vi "EOL Digital IO Status.vi"() -> ()   [LabVIEW 2018]
uses:
  05.UserVI's/type defs/EOL Global Digital Output Cluster Control.ctl
  05.UserVI's/type defs/EOL Global Digital Output Control.ctl
  05.UserVI's/type defs/EOL Global Digital Input Control.ctl
panel:
  in  "Tab Control":enum32{"Digital I/O", "RSLinx Tags"}(tab)
  out "Digital Inputs":T2(array[cluster])=[{"Status"=FALSE, "EOL Global Digital Input Control"=enum."Dev2/port0/line0"}, {"Status"=FALSE, "EOL Global Digital Input Control"=enum."Dev2/port0/line1"}, {"Status"=FALSE, "EOL Global Digital Input Control"=enum."Dev2/port0/line2"}, {"Status"=FALSE, "EOL Global Digital Input Control"=enum."Dev2/port0/line3"}, {"Status"=FALSE, "EOL Global Digital Input Control"=enum."Dev2/port0/line4"}, {"Status"=FALSE, "EOL Global Digital Input Control"=enum."Dev2/port0/line5"}, {"Status"=FALSE, "EOL Global Digital Input Control"=enum."Dev2/port0/line6"}, {"Status"=FALSE, "EOL Global Digital Input Control"=enum."Dev2/port0/line7"}, {"Status"=FALSE, "EOL Global Digital Input Control"=enum."Dev2/port1/line0"}, {"Status"=FALSE, "EOL Global Digital Input Control"=enum."Dev2/port1/line1"}, {"Status"=FALSE, "EOL Global Digital Input Control"=enum."Dev2/port1/line2"}, {"Status"=FALSE, "EOL Global Digital Input Control"=enum."Dev2/port1/line3"}, {"Status"=FALSE, "EOL Global Digital Input Control"=enum."Dev2/port1/line4"}, {"Status"=FALSE, "EOL Global Digital Input Control"=enum."Dev2/port1/line5"}, {"Status"=FALSE, "EOL Global Digital Input Control"=enum."Dev2/port1/line6"}, {"Status"=FALSE, "EOL Global Digital Input Control"=enum."Dev2/port1/line7"}, {"Status"=FALSE, "EOL Global Digital Input Control"=enum."Dev2/port2/line0"}, {"Status"=FALSE, "EOL Global Digital Input Control"=enum."Dev2/port2/line1"}, {"Status"=FALSE, "EOL Global Digital Input Control"=enum."Dev2/port2/line2"}, {"Status"=FALSE, "EOL Global Digital Input Control"=enum."Dev2/port2/line3"}, {"Status"=FALSE, "EOL Global Digital Input Control"=enum."Dev2/port2/line4"}, {"Status"=FALSE, "EOL Global Digital Input Control"=enum."Dev2/port2/line5"}, {"Status"=FALSE, "EOL Global Digital Input Control"=enum."Dev2/port2/line6"}, {"Status"=FALSE, "EOL Global Digital Input Control"=enum."Dev2/port2/line7"}, {"Status"=FALSE, "EOL Global Digital Input Control"=enum."Prerun Start Test"}, {"Status"=FALSE, "EOL Global Digital Input Control"=enum."Prerun Abort Test"}, {"Status"=FALSE, "EOL Global Digital Input Control"=enum."Audit Start Test"}, {"Status"=FALSE, "EOL Global Digital Input Control"=enum."Audit Abort Test"}, {"Status"=FALSE, "EOL Global Digital Input Control"=enum."Dev2/port3/line4"}, {"Status"=FALSE, "EOL Global Digital Input Control"=enum."Dev2/port3/line5"}, {"Status"=FALSE, "EOL Global Digital Input Control"=enum."Breakin Start Test"}, {"Status"=FALSE, "EOL Global Digital Input Control"=enum."Breakin Abort Test"}]
  out "Digital Output Status":T3[](array[typedef])=[{"Status"=FALSE, "Global DO Ch"=enum."Battery"}, {"Status"=FALSE, "Global DO Ch"=enum."Battery"}, {"Status"=FALSE, "Global DO Ch"=enum."Battery"}, {"Status"=FALSE, "Global DO Ch"=enum."Battery"}, {"Status"=FALSE, "Global DO Ch"=enum."Battery"}, {"Status"=FALSE, "Global DO Ch"=enum."Battery"}, {"Status"=FALSE, "Global DO Ch"=enum."Battery"}, {"Status"=FALSE, "Global DO Ch"=enum."Battery"}, {"Status"=FALSE, "Global DO Ch"=enum."Battery"}, {"Status"=FALSE, "Global DO Ch"=enum."Battery"}, {"Status"=FALSE, "Global DO Ch"=enum."Battery"}, {"Status"=FALSE, "Global DO Ch"=enum."Battery"}, {"Status"=FALSE, "Global DO Ch"=enum."Battery"}, {"Status"=FALSE, "Global DO Ch"=enum."Battery"}, {"Status"=FALSE, "Global DO Ch"=enum."Battery"}, {"Status"=FALSE, "Global DO Ch"=enum."Battery"}, {"Status"=FALSE, "Global DO Ch"=enum."Battery"}, {"Status"=FALSE, "Global DO Ch"=enum."Battery"}, {"Status"=FALSE, "Global DO Ch"=enum."Battery"}, {"Status"=FALSE, "Global DO Ch"=enum."Battery"}, {"Status"=FALSE, "Global DO Ch"=enum."Battery"}, {"Status"=FALSE, "Global DO Ch"=enum."Battery"}, {"Status"=FALSE, "Global DO Ch"=enum."Battery"}, {"Status"=FALSE, "Global DO Ch"=enum."Battery"}, {"Status"=FALSE, "Global DO Ch"=enum."Battery"}, {"Status"=FALSE, "Global DO Ch"=enum."Battery"}, {"Status"=FALSE, "Global DO Ch"=enum."Battery"}, {"Status"=FALSE, "Global DO Ch"=enum."Battery"}, {"Status"=FALSE, "Global DO Ch"=enum."Battery"}, {"Status"=FALSE, "Global DO Ch"=enum."Battery"}, {"Status"=FALSE, "Global DO Ch"=enum."Battery"}, {"Status"=FALSE, "Global DO Ch"=enum."Battery"}, {"Status"=FALSE, "Global DO Ch"=enum."Battery"}, {"Status"=FALSE, "Global DO Ch"=enum."Battery"}, {"Status"=FALSE, "Global DO Ch"=enum."Battery"}, {"Status"=FALSE, "Global DO Ch"=enum."Battery"}, {"Status"=FALSE, "Global DO Ch"=enum."Battery"}, {"Status"=FALSE, "Global DO Ch"=enum."Battery"}, {"Status"=FALSE, "Global DO Ch"=enum."Battery"}, {"Status"=FALSE, "Global DO Ch"=enum."Battery"}, {"Status"=FALSE, "Global DO Ch"=enum."Battery"}, {"Status"=FALSE, "Global DO Ch"=enum."Battery"}, {"Status"=FALSE, "Global DO Ch"=enum."Battery"}, {"Status"=FALSE, "Global DO Ch"=enum."Battery"}, {"Status"=FALSE, "Global DO Ch"=enum."Battery"}, {"Status"=FALSE, "Global DO Ch"=enum."Battery"}, {"Status"=FALSE, "Global DO Ch"=enum."Battery"}, {"Status"=FALSE, "Global DO Ch"=enum."Battery"}, {"Status"=FALSE, "Global DO Ch"=enum."Battery"}, {"Status"=FALSE, "Global DO Ch"=enum."Battery"}, {"Status"=FALSE, "Global DO Ch"=enum."Battery"}, {"Status"=FALSE, "Global DO Ch"=enum."Battery"}, {"Status"=FALSE, "Global DO Ch"=enum."Battery"}, {"Status"=FALSE, "Global DO Ch"=enum."Battery"}, {"Status"=FALSE, "Global DO Ch"=enum."Battery"}, {"Status"=FALSE, "Global DO Ch"=enum."Battery"}, {"Status"=FALSE, "Global DO Ch"=enum."Battery"}, {"Status"=FALSE, "Global DO Ch"=enum."Battery"}, {"Status"=FALSE, "Global DO Ch"=enum."Battery"}, {"Status"=FALSE, "Global DO Ch"=enum."Battery"}, {"Status"=FALSE, "Global DO Ch"=enum."Battery"}, {"Status"=FALSE, "Global DO Ch"=enum."Battery"}, {"Status"=FALSE, "Global DO Ch"=enum."Battery"}, {"Status"=FALSE, "Global DO Ch"=enum."Battery"}, {"Status"=FALSE, "Global DO Ch"=enum."Battery"}, {"Status"=FALSE, "Global DO Ch"=enum."Battery"}, {"Status"=FALSE, "Global DO Ch"=enum."Battery"}, {"Status"=FALSE, "Global DO Ch"=enum."Battery"}, {"Status"=FALSE, "Global DO Ch"=enum."Battery"}, {"Status"=FALSE, "Global DO Ch"=enum."Battery"}, {"Status"=FALSE, "Global DO Ch"=enum."Battery"}, {"Status"=FALSE, "Global DO Ch"=enum."Battery"}, {"Status"=FALSE, "Global DO Ch"=enum."Battery"}, {"Status"=FALSE, "Global DO Ch"=enum."Battery"}, {"Status"=FALSE, "Global DO Ch"=enum."Battery"}, {"Status"=FALSE, "Global DO Ch"=enum."Battery"}, {"Status"=FALSE, "Global DO Ch"=enum."Battery"}, {"Status"=FALSE, "Global DO Ch"=enum."Battery"}, {"Status"=FALSE, "Global DO Ch"=enum."Battery"}, {"Status"=FALSE, "Global DO Ch"=enum."Battery"}, {"Status"=FALSE, "Global DO Ch"=enum."Battery"}, {"Status"=FALSE, "Global DO Ch"=enum."Battery"}, {"Status"=FALSE, "Global DO Ch"=enum."Battery"}, {"Status"=FALSE, "Global DO Ch"=enum."Battery"}, {"Status"=FALSE, "Global DO Ch"=enum."Battery"}, {"Status"=FALSE, "Global DO Ch"=enum."Battery"}, {"Status"=FALSE, "Global DO Ch"=enum."Battery"}, {"Status"=FALSE, "Global DO Ch"=enum."Battery"}, {"Status"=FALSE, "Global DO Ch"=enum."Battery"}, {"Status"=FALSE, "Global DO Ch"=enum."Battery"}, {"Status"=FALSE, "Global DO Ch"=enum."Battery"}, {"Status"=FALSE, "Global DO Ch"=enum."Battery"}, {"Status"=FALSE, "Global DO Ch"=enum."Battery"}, {"Status"=FALSE, "Global DO Ch"=enum."Battery"}, {"Status"=FALSE, "Global DO Ch"=enum."Battery"}, {"Status"=FALSE, "Global DO Ch"=enum."Battery"}, {"Status"=FALSE, "Global DO Ch"=enum."Battery"}, {"Status"=FALSE, "Global DO Ch"=enum."Battery"}, {"Status"=FALSE, "Global DO Ch"=enum."Battery"}, {"Status"=FALSE, "Global DO Ch"=enum."Battery"}, {"Status"=FALSE, "Global DO Ch"=enum."Battery"}, {"Status"=FALSE, "Global DO Ch"=enum."Battery"}, {"Status"=FALSE, "Global DO Ch"=enum."Battery"}, {"Status"=FALSE, "Global DO Ch"=enum."Battery"}, {"Status"=FALSE, "Global DO Ch"=enum."Battery"}, {"Status"=FALSE, "Global DO Ch"=enum."Battery"}, {"Status"=FALSE, "Global DO Ch"=enum."Battery"}, {"Status"=FALSE, "Global DO Ch"=enum."Battery"}, {"Status"=FALSE, "Global DO Ch"=enum."Battery"}, {"Status"=FALSE, "Global DO Ch"=enum."Battery"}, {"Status"=FALSE, "Global DO Ch"=enum."Battery"}, {"Status"=FALSE, "Global DO Ch"=enum."Battery"}, {"Status"=FALSE, "Global DO Ch"=enum."Battery"}, {"Status"=FALSE, "Global DO Ch"=enum."Battery"}, {"Status"=FALSE, "Global DO Ch"=enum."Battery"}, {"Status"=FALSE, "Global DO Ch"=enum."Battery"}, {"Status"=FALSE, "Global DO Ch"=enum."Battery"}, {"Status"=FALSE, "Global DO Ch"=enum."Battery"}, {"Status"=FALSE, "Global DO Ch"=enum."Battery"}, {"Status"=FALSE, "Global DO Ch"=enum."Battery"}, {"Status"=FALSE, "Global DO Ch"=enum."Battery"}, {"Status"=FALSE, "Global DO Ch"=enum."Battery"}, {"Status"=FALSE, "Global DO Ch"=enum."Battery"}, {"Status"=FALSE, "Global DO Ch"=enum."Battery"}, {"Status"=FALSE, "Global DO Ch"=enum."Battery"}, {"Status"=FALSE, "Global DO Ch"=enum."Battery"}, {"Status"=FALSE, "Global DO Ch"=enum."Battery"}, {"Status"=FALSE, "Global DO Ch"=enum."Battery"}]
  out "RSLinx Read String":cluster{"Tag String":string, "String":string}[](array[cluster])
  out "RSLinx Read Boolean":cluster{"Tag String":string, "Boolean":bool}[](array[cluster])
  in  "Exit":bool
  # "Digital I/O Status"
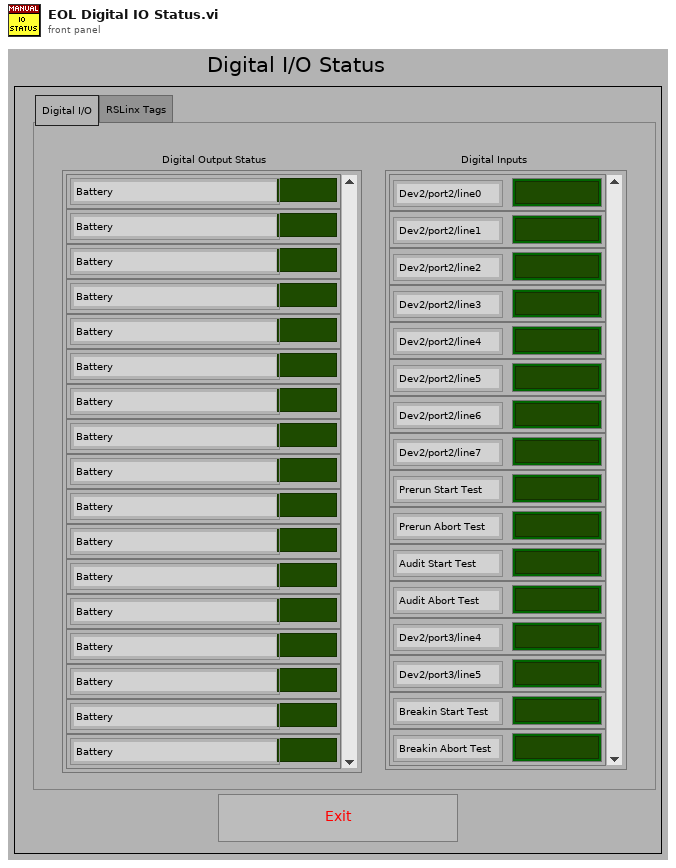
[diagram p1: front panel]
types:
  T1 = typedef "EOL Global Digital Input Control.ctl" = enum16{"Dev2/port0/line0", "Dev2/port0/line1", "Dev2/port0/line2", "Dev2/port0/line3", "Dev2/port0/line4", "Dev2/port0/line5", "Dev2/port0/line6", "Dev2/port0/line7", "Dev2/port1/line0", "Dev2/port1/line1", "Dev2/port1/line2", "Dev2/port1/line3", "Dev2/port1/line4", "Dev2/port1/line5", "Dev2/port1/line6", "Dev2/port1/line7", "Dev2/port2/line0", "Dev2/port2/line1", "Dev2/port2/line2", "Dev2/port2/line3", "Dev2/port2/line4", "Dev2/port2/line5", "Dev2/port2/line6", "Dev2/port2/line7", "Prerun Start Test", "Prerun Abort Test", "Audit Start Test", "Audit Abort Test", "Dev2/port3/line4", "Dev2/port3/line5", "Breakin Start Test", "Breakin Abort Test", "Not Implemented"}
  T2 = cluster{"Status":bool, "EOL Global Digital Input Control":T1}[]
  T3 = typedef "EOL Global Digital Output Cluster Control.ctl" = cluster{"Status":bool, "Global DO Ch":T4}
  T4 = typedef "EOL Global Digital Output Control.ctl" = enum16{"Battery", "IGN High", "IGN Low", "LIN", "CAN", "Switch 1", "Switch 2", "Switch 3", "Switch 4", "Switch 5", "Switch 6", "Glass Analog Switch 1", "Glass Analog Switch 2", "Glass Analog Switch 3", "Glass Analog Switch 4", "Sunshade Analog Switch 1", "Sunshade Analog Switch 2", "Sunshade Analog Switch 3", "Sunshade Analog Switch 4", "Glass Motor Relay 1", "Glass Motor Relay 2", "Sunshade Motor Relay 1", "Sunshade Motor Relay 2"}
  T5 = cluster{"RSLinx Write Boolean Names":string[], "RSLinx Write Boolean Tags":i32[], "RSLinx Write String Names":string[], "RSLinx Write String Tags":i32[], "RSLinx Read Boolean Names":string[], "RSLinx Read Boolean Tags":i32[], "RSLinx Read String Names":string[], "RSLinx Read String Tags":i32[], "Digital Output Array":T3[]}
  T6 = enum16{"Init", "Write", "Write All", "Clear All", "Stop", "Read"}
  T7 = cluster{"Status":bool, "EOL Global Digital Input Control":T1}
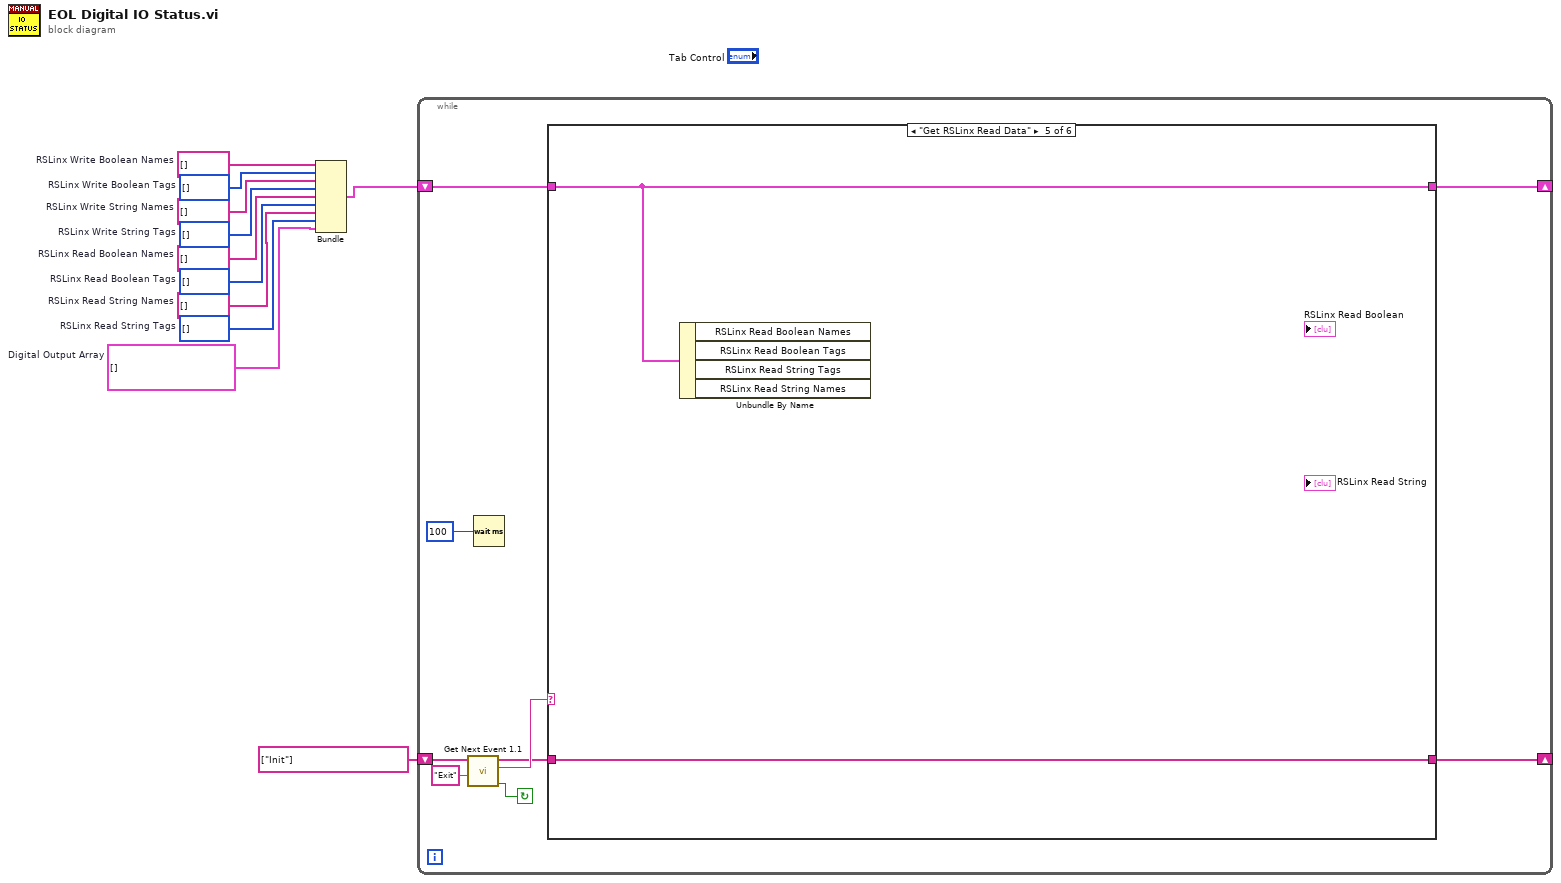
[diagram p0: block diagram]
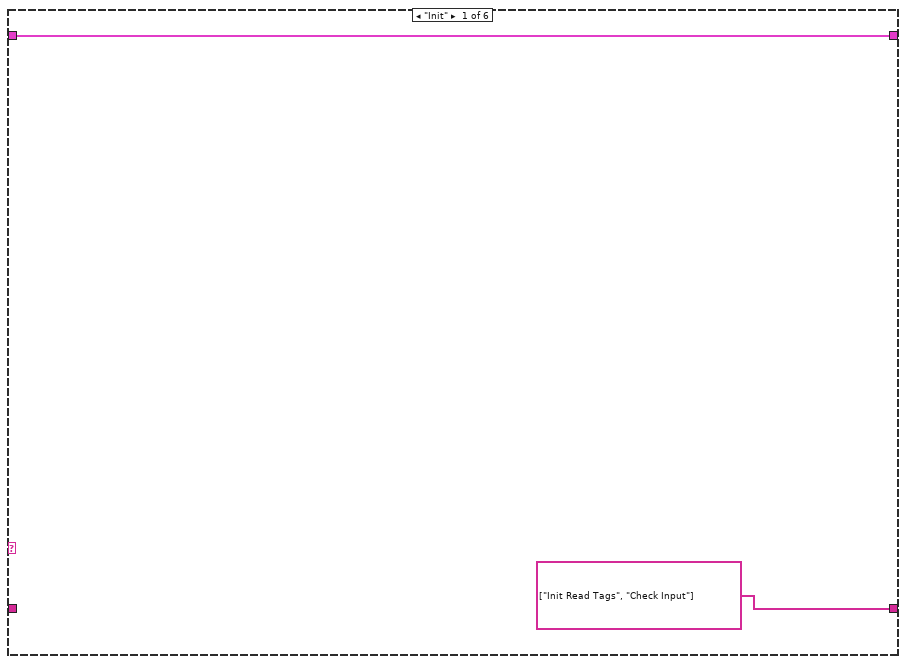
[diagram p2: hidden frame]
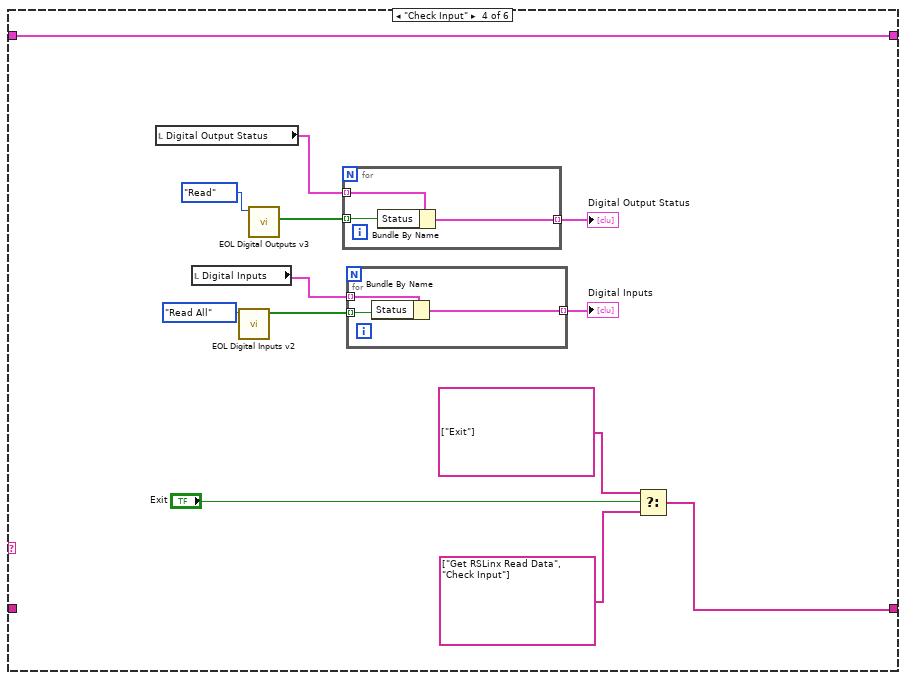
[diagram p5: hidden frame]
diagram:
  w1 = T3[] []  # Digital Output Array
  w5 = string[] []  # RSLinx Read String Names
  w4 = i32[] []  # RSLinx Read String Tags
  w7 = string[] []  # RSLinx Read Boolean Names
  w6 = i32[] []  # RSLinx Read Boolean Tags
  w9 = string[] []  # RSLinx Write String Names
  w8 = i32[] []  # RSLinx Write String Tags
  w11 = string[] []  # RSLinx Write Boolean Names
  w10 = i32[] []  # RSLinx Write Boolean Tags
  n1 = Bundle("RSLinx Write Boolean Names"=w11, "RSLinx Write Boolean Tags"=w10, "RSLinx Write String Names"=w9, "RSLinx Write String Tags"=w8, "RSLinx Read Boolean Names"=w7, "RSLinx Read Boolean Tags"=w6, "RSLinx Read String Names"=w5, "RSLinx Read String Tags"=w4, "Digital Output Array"=w1) -> (w3:T5)  [unwired: 1 in]
  n2 = while {
    shift-right: [w18] -> _
    shift-left: w3 -> [w19]
    shift-right: [w14] -> _
    shift-left: string[] ["Init"] ("event queue out") -> [w13]
    stop <- w12 continue-if-true
    n3 = call "Get Next Event 1.1.vi"("Exit Event"="Exit", "event queue in"=w13) -> ("Condition (Exit:F)"=w12:bool, "next event"=w16:string, "event queue out"=w15:string[])  [unwired: 6 in, 1 out]
    n4 = Wait (ms)(milliseconds to wait=u32 100) -> ()  [unwired: 1 out]
    n5 = case shown="\"Get RSLinx Read Data\"" w16 {
      tunnel: w19 -> [w22 w23 w25 w34 w47 w49]
      tunnel: [w22 w23 w25 w34 w47 w49] -> w18
      tunnel: w15 -> [_ w24 w26 _ w46 w48]
      tunnel: [string[] ["Init Read Tags", "Check Input"] ("event queue out") w24 w26 w27 w46 w48] -> w14
      frame "Init" {
      }
      frame "Init Read Tags" {
      }
      frame "Init Write Tags" {
      }
      frame "Check Input" {
        n6 = local read "Digital Output Status"() -> (w33:T3[])
        n7 = local read "Digital Inputs"() -> (w31:T2)
        n8 = call "EOL Digital Inputs v2.vi"("Mode"=enum16{"Init", "Read", "Read All", "Close"}."Read All") -> ("DI Status"=w36:bool[])  [unwired: 8 in, 2 out]
        n9 = call "EOL Digital Outputs v3.vi"("Mode"=T6."Read") -> ("Digital Out State 1"=w37:bool[])  [unwired: 9 in, 1 out]
        n10 = for {
          tunnel: w37 -> [w45] mode=indexing
          tunnel: w33 -> [w44] mode=indexing
          tunnel: [w43] -> w32 mode=indexing
          n11 = Bundle By Name(cluster=w44, "Status"=w45) -> (w43:T3)
        }
        "Digital Output Status" <- w32
        n12 = for {
          tunnel: w36 -> [w42] mode=indexing
          tunnel: w31 -> [w41] mode=indexing
          tunnel: [w40] -> w35 mode=indexing
          n13 = Bundle By Name(cluster=w41, "Status"=w42) -> (w40:T7)
        }
        "Digital Inputs" <- w35
        n14 = Select(t=string[] ["Exit"] ("event queue out"), s="Exit", f=string[] ["Get RSLinx Read Data", "Check Input"] ("event queue out")) -> (s? t:f=w27:string[])
      }
      frame "Get RSLinx Read Data" {
        n15 = Unbundle By Name(w47) -> ()  [unwired: 4 out]
      }
      frame "Exit", Default {
      }
    }
  }
